vi "3D_Line_v2.0.vi"() -> ()   [LabVIEW 2018]
uses:
  <vilib>/Native 3D Graph/xcontrol/3DPC_SurfacePlot.xctl
panel:
  out "3D Graph":refnum<class "Base Datatype.lvclass">[](xcontrol)
  out "Y":dbl format="%#.8g"
  out "Z":dbl
  out "X":dbl
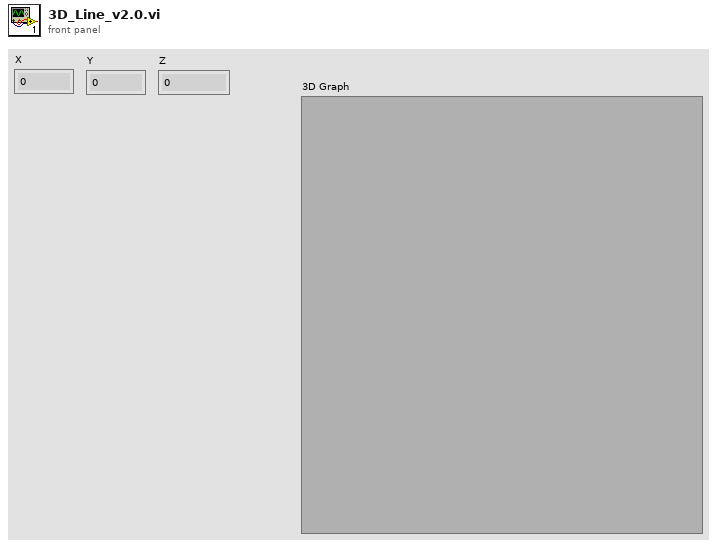
[diagram p1: front panel]
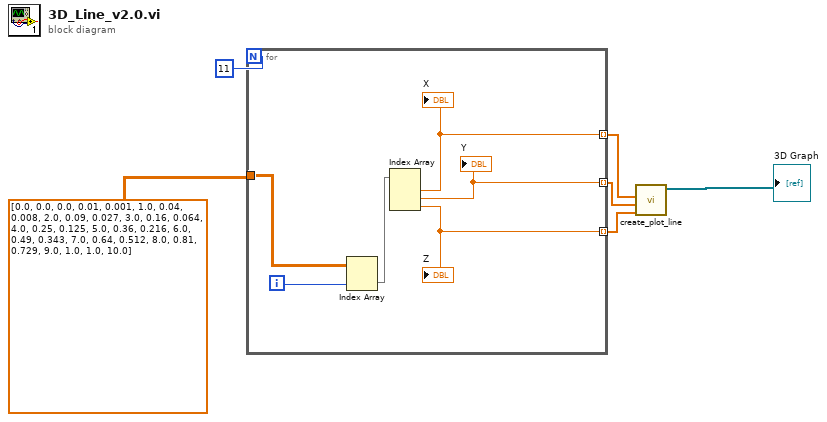
[diagram p0: block diagram]
diagram:
  n1 = for {
    N: 11 -> [_]
    tunnel: dbl[][] [[0.0, 0.0, 0.0], [0.01, 0.001, 1.0], [0.04, 0.008, 2.0], [0.09, 0.027, 3.0], [0.16, 0.064, 4.0], [0.25, 0.125, 5.0], [0.36, 0.216, 6.0], [0.49, 0.343, 7.0], [0.64, 0.512, 8.0], [0.81, 0.729, 9.0], [1.0, 1.0, 10.0]] ("Array") -> [w10]
    tunnel: [w9] -> w2 mode=indexing
    tunnel: [w8] -> w3 mode=indexing
    tunnel: [w7] -> w4 mode=indexing
    i -> [w12]
    n2 = Index Array(array=w10, index (row)=w12) -> (element=w11:dbl[])  [unwired: 1 in]
    n3 = Index Array(array=w11) -> (element #1=w9:dbl, element #2=w8:dbl, element #3=w7:dbl)  [unwired: 3 in]
    "Y" <- w8
    "Z" <- w7
    "X" <- w9
  }
  n4 = call <vilib>:"create_plot_line.vi"("z vector"=w4, "y vector"=w3, "x vector"=w2) -> ("plots out"=→"3D Graph":refnum<class "Base Datatype.lvclass">[])  [unwired: 2 in, 6 out]
